vi "Sequencer Main.vi"() -> ()   [LabVIEW 2018] (continued)
              n174 = Greater Than 0?(x=w225) -> (x > 0?=w228:bool)
              n175 = case shown="True" w228 {
                tunnel: w225 -> [_ w233]
                tunnel: [0 w232] -> w227
                frame False {
                }
                frame True {
                  n176 = Decrement(x=w233) -> (x-1=w232:i32)
                }
              }
              n177 = Initialize Array(0, w225) -> (w223:i32[])
              n178 = Greater?(x=w226, y=w227) -> (0:w230:bool)
              n179 = case shown="True" w230 {
                tunnel: w227 -> [_ w235]
                tunnel: w226 -> [w234 _]
                frame False {
                  n180 = local write "Break Point Line"(w234) -> ()
                  n181 = property on="Test Sequencer" class="MCListbox (strict)"("Value"=w234) -> ()  [unwired: 2 in, 2 out]
                }
                frame True {
                  n182 = local write "Break Point Line"(w235) -> ()
                  n183 = property on="Test Sequencer" class="MCListbox (strict)"("Value"=w235) -> ()  [unwired: 2 in, 2 out]
                }
              }
            }
            frame #1 {
              n184 = local read "Break Point Line"() -> (w238:u32)
              n185 = Replace Array Subset(array=w237, new element=1 ("new element/subarray"), index=w238) -> (w239:i32[])
              n186 = global write "Global Variable.vi" "Simbol Array"(w239) -> ()
              n187 = property on="Test Sequencer" class="MCListbox (strict)"("ItemSyms"=w239) -> ()  [unwired: 2 in, 2 out]
            }
          }
        }
        event "Break Point Line": Value Change {
          n188 = event-data() -> ("NewVal"=w241:u32)  [unwired: 1 in, 5 out]
          n189 = flat-sequence {
            tunnel: w241 -> [w245]
            tunnel: [w242] -> w240
            tunnel: w240 -> [w256]
            frame #0 {
              n190 = global read "Sequencer Array.vi" "SEQUENCER Array"() -> (w248:T16[])
              n191 = Array Size(array=w248) -> (size(s)=w244:i32)
              n192 = Greater Than 0?(x=w244) -> (x > 0?=w247:bool)
              n193 = case shown="True" w247 {
                tunnel: w244 -> [_ w252]
                tunnel: [0 w251] -> w246
                frame False {
                }
                frame True {
                  n194 = Decrement(x=w252) -> (x-1=w251:i32)
                }
              }
              n195 = Initialize Array(0, w244) -> (w242:i32[])
              n196 = Greater?(x=w245, y=w246) -> (0:w249:bool)
              n197 = case shown="True" w249 {
                tunnel: w246 -> [_ w254]
                tunnel: w245 -> [w253 _]
                frame False {
                  n198 = local write "Break Point Line"(w253) -> ()
                  n199 = property on="Test Sequencer" class="MCListbox (strict)"("Value"=w253) -> ()  [unwired: 2 in, 2 out]
                }
                frame True {
                  n200 = local write "Break Point Line"(w254) -> ()
                  n201 = property on="Test Sequencer" class="MCListbox (strict)"("Value"=w254) -> ()  [unwired: 2 in, 2 out]
                }
              }
            }
            frame #1 {
              n202 = local read "Break Point Line"() -> (w257:u32)
              n203 = Replace Array Subset(array=w256, new element=1 ("new element/subarray"), index=w257) -> (w258:i32[])
              n204 = global write "Global Variable.vi" "Simbol Array"(w258) -> ()
              n205 = property on="Test Sequencer" class="MCListbox (strict)"("ItemSyms"=w258) -> ()  [unwired: 2 in, 2 out]
            }
          }
        }
        event "Abort Test": Value Change {
          n206 = event-data() -> ()  [unwired: 1 in, 6 out]
          n207 = local read "Debugging"() -> (w261:bool)
          n208 = case shown="True" w261 {
            tunnel: w263 -> [w265 w282]
            tunnel: w262 -> [w266 w281]
            frame False {
              # "!!!!Test Steps Must-be more then 2"
              n209 = global read "Global Variable.vi" "Steps Nmb"() -> (w269:u32)
              n210 = Greater Or Equal?(x=w269, y=u32 2) -> (x >= y?=w268:bool)
              n211 = case shown="True" w268 {
                tunnel: w266 -> [_ w277]
                tunnel: w265 -> [_ w276]
                frame False {
                }
                frame True {
                  w273 = T14 {"Row"=0, "Column"=0} ("Top Left Visible Cell")
                  n212 = global read "Global Variable.vi" "Steps Nmb"() -> (w272:u32)
                  n213 = Subtract(x=w272, y=u32 1) -> (x-y=w271:u32)
                  n214 = Flush Queue(queue=w276, error in (no error)=w277) -> (queue out=w279:refnum<queue>, error out=w278:errorcluster)  [unwired: 1 out]
                  n215 = Enqueue Element(queue=w279, element=w271, error in (no error)=w278) -> ()  [unwired: 1 in, 3 out]
                  n216 = global read "Global Variable.vi" "Report Step Nmb"() -> (w270:u32)
                  n217 = Bundle By Name(cluster=w273, "Row"=w271) -> (w275:T14)
                  n218 = Bundle By Name(cluster=w273, "Row"=w270) -> (w274:T14)
                  n219 = property on="Test Sequencer Run" class="MCListbox (strict)"("TopLeft"=w274) -> ()  [unwired: 2 in, 2 out]
                  n220 = property on="Test Sequencer" class="MCListbox (strict)"("TopLeft"=w275) -> ()  [unwired: 2 in, 2 out]
                }
              }
              n221 = local read "Auto\nRestart"() -> (w264:u16)
              n222 = local write "Restart Cnt"(w264) -> ()
            }
            frame True {
              n223 = flat-sequence {
                tunnel: w282 -> [w290]
                tunnel: w281 -> [w289]
                frame #0 {
                  n224 = global read "Global Variable.vi" "Steps Nmb"() -> (w286:u32)
                  n225 = global read "Global Variable.vi" "Current Step Nmb"() -> (w284:u32)
                  n226 = Decrement(x=w286) -> (x-1=w285:u32)
                  n227 = Greater?(x=w285, y=w284) -> (0:w283:bool)
                  n228 = case shown="True" w283 {
                    frame False {
                    }
                    frame True {
                      n229 = local write "Message"("!!! TEST ABORTED By USER" ("Message")) -> ()
                    }
                  }
                }
                frame #1 {
                  n230 = global read "Global Variable.vi" "Steps Nmb"() -> (w293:u32)
                  n231 = Flush Queue(queue=w290, error in (no error)=w289) -> (queue out=w291:refnum<queue>, error out=w292:errorcluster)  [unwired: 1 out]
                  n232 = local read "Auto\nRestart"() -> (w288:u16)
                  n233 = Decrement(x=w293) -> (x-1=w294:u32)
                  n234 = Enqueue Element(queue=w291, element=w294, error in (no error)=w292) -> ()  [unwired: 1 in, 3 out]
                  n235 = global write "Global Variable.vi" "Current Step Nmb"(w294) -> ()
                  n236 = local write "Restart Cnt"(w288) -> ()
                }
              }
            }
          }
          n237 = global write "Global Variable.vi" "Test Gen Status"(FALSE ("Test Gen Status")) -> ()
          n238 = global write "Global Variable.vi" "System Status"(T1."STOP Sequencer" ("System Status")) -> ()
        }
        event "Load Sequenser": Value Change {
          n239 = event-data() -> ()  [unwired: 1 in, 6 out]
          n240 = global write "Global Variable.vi" "Active Lines Cnt"(u32 0 ("Active Lines Cnt")) -> ()
          n241 = global write "Global Variable.vi" "Report Step Nmb"(u32 0 ("Report Step Nmb")) -> ()
          n242 = control-ref of="Test Sequencer"() -> (w297:refnum<vi>)
          n243 = property on="Tab Edit/Run" class="TabCtl (strict)"("Value"=enum32{"Edit", "Run"}."Edit" ("Tab Edit/Run")) -> ()  [unwired: 2 in, 2 out]
          n244 = in-place {
            in-place-border: w297 -> [w326]
            # "Set Color of all Row to White (Devices)"
            n245 = for {
              N: 250 -> [_]
              tunnel: w326 -> [w328]
              i -> [w329]
              n246 = for {
                N: 10 -> [_]
                tunnel: w329 -> [w334]
                tunnel: w328 -> [w331]
                i -> [w335]
                n247 = Bundle By Name(cluster=T15 {"Row"=0, "Column"=0} ("Active Cell:Active Cell"), "Row"=w334, "Column"=w335) -> (w333:T15)
                n248 = property on="Property Node" class="MCListbox (strict)"(reference=w331, "ActiveCell"=w333, "CellBG"=u32 14013909) -> ()  [unwired: 1 in, 2 out]
              }
            }
          }
          n249 = in-place "In Place Element Structure" {
            in-place-border: w297 -> [w319]
            # "Cleare Sequencer Table"
            n250 = Initialize Array("", 250 ("dimension size"), 10 ("dimension size")) -> (w323:string[][])
            n251 = property on="Property Node" class="MCListbox (strict)"(reference=w319, "ItemNames"=w323, "TopLeft"=T14 {"Row"=0, "Column"=0} ("Top Left Visible Cell"), "Value"=T11 0 ("Test Sequencer")) -> ()  [unwired: 1 in, 2 out]
          }
          n252 = control-ref of="Test Sequencer Run"() -> (w296:refnum<vi>)
          n253 = in-place {
            in-place-border: w296 -> [w308]
            # "Set Color of all Row on Report Table"
            n254 = for {
              N: 250 -> [_]
              tunnel: w308 -> [w310]
              i -> [w311]
              n255 = for {
                N: 7 -> [_]
                tunnel: w311 -> [w316]
                tunnel: w310 -> [w313]
                i -> [w317]
                n256 = Bundle By Name(cluster=T15 {"Row"=0, "Column"=0} ("Active Cell:Active Cell"), "Row"=w316, "Column"=w317) -> (w315:T15)
                n257 = property on="Property Node" class="MCListbox (strict)"(reference=w313, "ActiveCell"=w315, "CellBG"=u32 16448250) -> ()  [unwired: 1 in, 2 out]
              }
            }
          }
          n258 = in-place "In Place Element Structure" {
            in-place-border: w296 -> [w301]
            # "Cleare Sequencer Report Table"
            n259 = Initialize Array("", 250 ("dimension size"), 7 ("dimension size")) -> (w305:string[][])
            n260 = property on="Property Node" class="MCListbox (strict)"(reference=w301, "ItemNames"=w305, "TopLeft"=T14 {"Row"=0, "Column"=0} ("Top Left Visible Cell"), "Value"=T11 0 ("Test Sequencer")) -> ()  [unwired: 1 in, 2 out]
          }
          n261 = global write "Global Variable.vi" "System Status"(T1."INI Secuencer" ("System Status")) -> ()
        }
        event "Button Next Step": Value Change {
          n262 = event-data() -> ()  [unwired: 1 in, 6 out]
          n263 = global read "Global Variable.vi" "Steps Nmb"() -> (w341:u32)
          n264 = global read "Global Variable.vi" "Current Step Nmb"() -> (w340:u32)
          n265 = Decrement(x=w341) -> (x-1=w339:u32)
          n266 = Equal?(x=w339, y=w340) -> (x = y?=w342:bool)
          n267 = case shown="False" w342 {
            tunnel: w338 -> [w345 _]
            tunnel: w337 -> [w344 _]
            frame False {
              n268 = global read "Global Variable.vi" "Current Step Nmb"() -> (w349:u32)
              n269 = Flush Queue(queue=w345, error in (no error)=w344) -> (queue out=w348:refnum<queue>, error out=w347:errorcluster)  [unwired: 1 out]
              n270 = Increment(x=w349) -> (x+1=w346:u32)
              n271 = global write "Global Variable.vi" "Current Step Nmb"(w346) -> ()
              n272 = Enqueue Element(queue=w348, element=w346, error in (no error)=w347) -> ()  [unwired: 1 in, 3 out]
              n273 = global write "Global Variable.vi" "System Status"(T1."START Sequencer" ("System Status")) -> ()
            }
            frame True {
              n274 = global write "Global Variable.vi" "System Status"(T1."Idle" ("System Status")) -> ()
            }
          }
        }
        event "Button Retest": Value Change {
          n275 = event-data() -> ()  [unwired: 1 in, 6 out]
          n276 = global read "Global Variable.vi" "Steps Nmb"() -> (w355:u32)
          n277 = global read "Global Variable.vi" "Current Step Nmb"() -> (w354:u32)
          n278 = Decrement(x=w355) -> (x-1=w353:u32)
          n279 = Equal?(x=w353, y=w354) -> (x = y?=w356:bool)
          n280 = case shown="False" w356 {
            tunnel: w352 -> [w360 _]
            tunnel: w351 -> [w359 _]
            frame False {
              n281 = global read "Global Variable.vi" "Current Step Nmb"() -> (w358:u32)
              n282 = Flush Queue(queue=w360, error in (no error)=w359) -> (queue out=w362:refnum<queue>, error out=w361:errorcluster)  [unwired: 1 out]
              n283 = global write "Global Variable.vi" "Current Step Nmb"(w358) -> ()
              n284 = Enqueue Element(queue=w362, element=w358, error in (no error)=w361) -> ()  [unwired: 1 in, 3 out]
              n285 = global write "Global Variable.vi" "System Status"(T1."START Sequencer" ("System Status")) -> ()
            }
            frame True {
              n286 = global write "Global Variable.vi" "System Status"(T1."Idle" ("System Status")) -> ()
            }
          }
        }
        event "Reset cnt": Value Change {
          w364 = 0
          n287 = event-data() -> ()  [unwired: 1 in, 6 out]
          n288 = local write "Cnt Total"(w364) -> ()
          n289 = local write "Cnt Pass"(w364) -> ()
          n290 = local write "Cnt False"(w364) -> ()
        }
        event "Sequenser": Value Change {
          n291 = event-data() -> ("NewVal"=w367:u16)  [unwired: 1 in, 5 out]
          n292 = global read "Global Variable.vi" "Sequencer Path"() -> (w368:path[])
          n293 = Index Array(array=w368, index=w367) -> (element=w365:path)
          n294 = call-poly <userlib>:"File Exists__ogtk.vi"("file path"=w365) -> ("exists"=w366:bool)  [unwired: 6 in, 1 out]
          n295 = case shown="True" w366 {
            tunnel: w365 -> [_ w372]
            frame False {
            }
            frame True {
              n296 = call <vilib>:"Set Busy.vi"() -> ("error out"=w371:errorcluster)  [unwired: 10 in, 1 out]
              n297 = flat-sequence {
                tunnel: w371 -> [w375]
                tunnel: [w375] -> w370
                tunnel: [w425] -> w374
                tunnel: [w424] -> w373
                tunnel: w372 -> [w422]
                tunnel: w370 -> [w421]
                tunnel: [w421] -> w369
                tunnel: w374 -> [w521]
                tunnel: w373 -> [w520]
                tunnel: w369 -> [w518]
                frame #0 {
                  n298 = global read "Sequencer Array.vi" "SEQUENCER Array"() -> (w378:T16[])
                  n299 = global write "Global Variable.vi" "Steps Cnt"(0) -> ()
                  n300 = control-ref of="Test Sequencer"() -> (w384:refnum<vi>)
                  n301 = global write "Global Variable.vi" "Active Lines Cnt"(u32 0 ("Active Lines Cnt")) -> ()
                  n302 = global write "Global Variable.vi" "Report Step Nmb"(u32 0 ("Report Step Nmb")) -> ()
                  n303 = property on="Tab Edit/Run" class="TabCtl (strict)"("Value"=enum32{"Edit", "Run"}."Edit" ("Tab Edit/Run")) -> ()  [unwired: 2 in, 2 out]
                  n304 = in-place {
                    in-place-border: w384 -> [w403]
                    # "Set Color of all Row to White (Devices)"
                    n305 = for {
                      N: 250 -> [_]
                      tunnel: w403 -> [w405]
                      i -> [w406]
                      n306 = for {
                        N: 10 -> [_]
                        tunnel: w406 -> [w411]
                        tunnel: w405 -> [w408]
                        i -> [w412]
                        n307 = Bundle By Name(cluster=T15 {"Row"=0, "Column"=0} ("Active Cell:Active Cell"), "Row"=w411, "Column"=w412) -> (w410:T15)
                        n308 = property on="Property Node" class="MCListbox (strict)"(reference=w408, "ActiveCell"=w410, "CellBG"=u32 14013909) -> ()  [unwired: 1 in, 2 out]
                      }
                    }
                  }
                  n309 = Array Size(array=w378) -> (size(s)=w377:i32)
                  n310 = in-place "In Place Element Structure" {
                    in-place-border: w384 -> [w414]
                    # "Cleare Sequencer Table"
                    n311 = Initialize Array("", 250 ("dimension size"), 10 ("dimension size")) -> (w418:string[][])
                    n312 = property on="Property Node" class="MCListbox (strict)"(reference=w414, "ItemNames"=w418, "TopLeft"=T14 {"Row"=0, "Column"=0} ("Top Left Visible Cell"), "Value"=T11 0 ("Test Sequencer")) -> ()  [unwired: 1 in, 2 out]
                  }
                  n313 = Delete From Array(array=w378, length=w377) -> (array with subset deleted=w376:T16[])  [unwired: 1 in, 1 out]
                  n314 = global write "Sequencer Array.vi" "SEQUENCER Array"(w376) -> ()
                  n315 = control-ref of="Test Sequencer Run"() -> (w380:refnum<vi>)
                  n316 = in-place "In Place Element Structure" {
                    in-place-border: w380 -> [w396]
                    # "Cleare Sequencer Report Table"
                    n317 = Initialize Array("", 250 ("dimension size"), 7 ("dimension size")) -> (w400:string[][])
                    n318 = property on="Property Node" class="MCListbox (strict)"(reference=w396, "ItemNames"=w400, "TopLeft"=T14 {"Row"=0, "Column"=0} ("Top Left Visible Cell"), "Value"=T11 0 ("Test Sequencer")) -> ()  [unwired: 1 in, 2 out]
                  }
                  n319 = in-place {
                    in-place-border: w380 -> [w385]
                    # "Set Color of all Row on Report Table"
                    n320 = for {
                      N: 250 -> [_]
                      tunnel: w385 -> [w387]
                      i -> [w388]
                      n321 = for {
                        N: 7 -> [_]
                        tunnel: w388 -> [w393]
                        tunnel: w387 -> [w390]
                        i -> [w394]
                        n322 = Bundle By Name(cluster=T15 {"Row"=0, "Column"=0} ("Active Cell:Active Cell"), "Row"=w393, "Column"=w394) -> (w392:T15)
                        n323 = property on="Property Node" class="MCListbox (strict)"(reference=w390, "ActiveCell"=w392, "CellBG"=u32 16448250) -> ()  [unwired: 1 in, 2 out]
                      }
                    }
                  }
                }
                frame #1 {
                  n324 = call <vilib>:"Open Config Data.vi"("create file if necessary (T)"=FALSE, "configuration file path"=w422) -> ("error out"=w429:errorcluster, "refnum"=w430:T19)  [unwired: 7 in, 1 out]
                  n325 = global write "Global Variable.vi" "Steps Cnt"(u16 0 ("Steps Cnt")) -> ()
                  n326 = call <vilib>:"Get Section Names.vi"("error in (no error)"=w429, "refnum"=w430) -> ("error out"=w427:errorcluster, "section names"=w428:string[], "refnum out"=w426:T19)  [unwired: 7 in]
                  n327 = for {
                    tunnel: w428 -> [w436] mode=indexing
                    tunnel: w427 -> [w441]
                    tunnel: w426 -> [w440]
                    tunnel: [w433] -> w425
                    tunnel: [w432] -> w424
                    n328 = Equal?(x=w436, y="Info") -> (x = y?=w442:bool)
                    n329 = case shown="True" w442 {
                      tunnel: w441 -> [w499 w505]
                      tunnel: w440 -> [w500 w504]
                      tunnel: [w500 w503] -> w435
                      tunnel: [w499 w502] -> w434
                      frame False {
                      }
                      frame True {
                        w516 = "***"
                        w512 = "Info"
                        n330 = call-poly <vilib>:"Read Key.vi"("section"=w512, "error in (no error)"=w505, "default value"=w516, "key"="Customer", "refnum"=w504) -> ("error out"=w509:errorcluster, "value"=w501:string, "refnum out"=w511:T19)  [unwired: 3 in, 1 out]
                        n331 = call-poly <vilib>:"Read Key.vi"("section"=w512, "error in (no error)"=w509, "default value"=w516, "key"="Board", "refnum"=w511) -> ("error out"=w508:errorcluster, "value"=w507:string, "refnum out"=w510:T19)  [unwired: 3 in, 1 out]
                        n332 = call-poly <vilib>:"Read Key.vi"("section"=w512, "error in (no error)"=w508, "default value"=w516, "key"="Config", "refnum"=w510) -> ("error out"=w502:errorcluster, "value"=w506:string, "refnum out"=w503:T19)  [unwired: 3 in, 1 out]
                        n333 = global write "Global Variable.vi" "Customer"(w501) -> ()
                        n334 = global write "Global Variable.vi" "Config"(w506) -> ()
                        n335 = global write "Global Variable.vi" "Board"(w507) -> ()
                      }
                    }
                    n336 = Match Pattern(string=w436, regular expression="Step") -> (offset past match=w439:i32)  [unwired: 1 in, 3 out]
                    n337 = Greater Or Equal To 0?(x=w439) -> (x >= 0?=w437:bool)
                    n338 = case shown="True" w437 {
                      tunnel: w436 -> [_ w463]
                      tunnel: w435 -> [w445 w462]
                      tunnel: w434 -> [w444 w461]
                      tunnel: [w445 w449] -> w433
                      tunnel: [w444 w448] -> w432
                      frame False {
                      }
                      frame True {
                        n339 = call-poly <vilib>:"Read Key.vi"("section"=w463, "error in (no error)"=w461, "key"="Step ID", "refnum"=w462) -> ("error out"=w466:errorcluster, "value"=w460:u32, "refnum out"=w465:T19)  [unwired: 4 in, 1 out]
                        n340 = call-poly <vilib>:"Read Key.vi"("section"=w463, "error in (no error)"=w466, "key"="Description", "refnum"=w465) -> ("error out"=w470:errorcluster, "value"=w459:string, "refnum out"=w469:T19)  [unwired: 4 in, 1 out]
                        n341 = call-poly <vilib>:"Read Key.vi"("section"=w463, "error in (no error)"=w470, "key"="Step Type", "refnum"=w469) -> ("error out"=w473:errorcluster, "value"=w458:u32, "refnum out"=w472:T19)  [unwired: 4 in, 1 out]
                        n342 = call-poly <vilib>:"Read Key.vi"("section"=w463, "error in (no error)"=w473, "key"="Measurement Units", "refnum"=w472) -> ("error out"=w477:errorcluster, "value"=w457:string, "refnum out"=w474:T19)  [unwired: 4 in, 1 out]
                        n343 = call-poly <vilib>:"Read Key.vi"("section"=w463, "error in (no error)"=w477, "key"="Nominal Value", "refnum"=w474) -> ("error out"=w478:errorcluster, "value"=w456:dbl, "refnum out"=w475:T19)  [unwired: 4 in, 1 out]
                        n344 = global read "Global Variable.vi" "Steps Cnt"() -> (w446:u16)
                        n345 = call-poly <vilib>:"Read Key.vi"("section"=w463, "error in (no error)"=w478, "key"="Upper Value", "refnum"=w475) -> ("error out"=w479:errorcluster, "value"=w455:dbl, "refnum out"=w476:T19)  [unwired: 4 in, 1 out]
                        n346 = Increment(x=w446) -> (x+1=w447:u16)
                        n347 = call-poly <vilib>:"Read Key.vi"("section"=w463, "error in (no error)"=w479, "key"="Lower Value", "refnum"=w476) -> ("error out"=w484:errorcluster, "value"=w454:dbl, "refnum out"=w483:T19)  [unwired: 4 in, 1 out]
                        n348 = global write "Global Variable.vi" "Steps Cnt"(w447) -> ()
                        n349 = call-poly <vilib>:"Read Key.vi"("section"=w463, "error in (no error)"=w484, "key"="Parameters", "refnum"=w483) -> ("error out"=w489:errorcluster, "value"=w453:string, "refnum out"=w486:T19)  [unwired: 4 in, 1 out]
                        n350 = call-poly <vilib>:"Read Key.vi"("section"=w463, "error in (no error)"=w489, "key"="Run/Skip", "refnum"=w486) -> ("error out"=w490:errorcluster, "value"=w452:bool, "refnum out"=w487:T19)  [unwired: 4 in, 1 out]
                        n351 = call-poly <vilib>:"Read Key.vi"("section"=w463, "error in (no error)"=w490, "key"="Report", "refnum"=w487) -> ("error out"=w491:errorcluster, "value"=w451:bool, "refnum out"=w488:T19)  [unwired: 4 in, 1 out]
                        n352 = call-poly <vilib>:"Read Key.vi"("section"=w463, "error in (no error)"=w491, "key"="Test Result", "refnum"=w488) -> ("error out"=w448:errorcluster, "value"=w450:u32, "refnum out"=w449:T19)  [unwired: 4 in, 1 out]
                        n353 = Bundle By Name(cluster=T16 {"Step ID"=0, "Step Description"="", "Step Type"=0, "Test Values"={"Numeric Value"=0.0, "Str Value"="", "Boolean Value"=TRUE, "Upper Limit"=0.0, "Lower Limit"=0.0}, "Parameters"="", "Run/Skip"=TRUE, "Test Result"=enum."Idle", "Report"=TRUE, "Measure Units"="..."} ("Test Step"), "Step ID"=w460, "Step Description"=w459, "Step Type"=w458, "Measure Units"=w457, "Test Values.Numeric Value"=w456, "Test Values.Upper Limit"=w455, "Test Values.Lower Limit"=w454, "Parameters"=w453, "Run/Skip"=w452, "Report"=w451, "Test Result"=w450) -> (w498:T16)
                        n354 = global read "Sequencer Array.vi" "SEQUENCER Array"() -> (w495:T16[])
                        n355 = Insert Into Array(array=w495, index=w446, new element=w498) -> (w496:T16[])
                        n356 = global write "Sequencer Array.vi" "SEQUENCER Array"(w496) -> ()
                      }
                    }
                  }
                }
                frame #2 {
                  n357 = in-place {
                    n358 = global write "Global Variable.vi" "System Status"(T1."INI Secuencer" ("System Status")) -> ()
                  }
                  n359 = call <vilib>:"Unset Busy.vi"("error in (no error)"=w518) -> ("error out"=w517:errorcluster)  [unwired: 10 in]
                  n360 = call <vilib>:"Close Config Data.vi"("error in (no error)"=w520, "write file if changed (T)"=TRUE, "refnum"=w521) -> ("error out"=w523:errorcluster)  [unwired: 7 in, 1 out]
                  n361 = call <userlib>:"Clear All Errors__ogtk.vi"("Error In"=w517) -> ()  [unwired: 3 in, 1 out]
                  n362 = call <vilib>:"Simple Error Handler.vi"("error in (no error)"=w523) -> ()  [unwired: 4 in, 5 out]
                  n363 = property on="Tab Control Main" class="TabCtl (strict)"("Value"=T2."TEST Board" ("Tab Control Main")) -> ()  [unwired: 2 in, 2 out]
                }
              }
            }
          }
        }
      }
    }
  }
  n364 = in-place {
    in-place-border: w5 -> [w528]
    in-place-border: w4 -> [w527]
    in-place-border: w3 -> [w526]
    in-place-border: w2 -> [w525]
    n365 = while {
      tunnel: w528 -> [w532]
      tunnel: w527 -> [w531]
      tunnel: w526 -> [w530]
      tunnel: w525 -> [w529]
      stop <- FALSE stop-if-true
      # "250"
      # "READ System GPIO"
      n366 = event shown="[0] Timeout" {
        selector: _ -> [_]
        dyn-events: _ -> [_]
        timeout: 50 -> [_]
        tunnel: w532 -> [w539]
        tunnel: w531 -> [w540]
        tunnel: w530 -> [w536]
        tunnel: w529 -> [w535]
        event Timeout {
          n367 = event-data() -> ()  [unwired: 1 in, 3 out]
          n368 = call <vilib>:"Acquire Semaphore.vi"("error in (no error)"=w539, "semaphore"=w540) -> ("error out"=w538:errorcluster, "semaphore out"=w537:T13)  [unwired: 3 in, 1 out]
          n369 = case shown="No Error" w538 {
            selector: w538 -> [w557 _]
            tunnel: w537 -> [w556 _]
            tunnel: w536 -> [w555 _]
            tunnel: w535 -> [w554 _]
            frame No Error {
              n370 = flat-sequence {
                tunnel: w557 -> [w559]
                tunnel: w556 -> [w558]
                tunnel: w555 -> [w588]
                tunnel: [w588] -> w553
                tunnel: w554 -> [w593]
                tunnel: [w593] -> w552
                tunnel: [w580] -> w551
                tunnel: [w578] -> w550
                tunnel: [w576] -> w549
                tunnel: [w575] -> w548
                tunnel: [w564] -> w543
                tunnel: [w559] -> w542
                tunnel: [w558] -> w541
                tunnel: w553 -> [w653]
                tunnel: [w653] -> w547
                tunnel: w552 -> [w652]
                tunnel: [w652] -> w546
                tunnel: [w649] -> w545
                tunnel: w551 -> [w650]
                tunnel: w550 -> [w644]
                tunnel: w549 -> [w645]
                tunnel: w548 -> [w651]
                tunnel: [w647] -> w544
                tunnel: w543 -> [w648]
                tunnel: w542 -> [w643]
                tunnel: w541 -> [w642]
                tunnel: w544 -> [w660]
                tunnel: w545 -> [w662]
                tunnel: w546 -> [w663]
                tunnel: w547 -> [w661]
                frame #0 {
                  w602 = T20 7 items=["Addr-0"=0, "Addr-1"=4, "Addr-2"=2, "Addr-3"=6, "Addr-4"=1, "Addr-5"=5, "Addr-6"=3, "Addr-7"=7] ("Addr")
                  # "DigIn 3"
                  # "ReSTART"
                  # "no dio err"
                  # "Stop AUTO"
                  # "Start AUTO"
                  # "Start Button"
                  # "Stop Button"
                  # "READ SYS Dig In"
                  n371 = global read "Global Variable.vi" "FTDI SPI Handle"() -> (w603:u32)
                  n372 = in-place {
                    in-place-border: [w631] -> _
                    in-place-border: [w630] -> w592
                    n373 = property on="Tab Control Main" class="TabCtl (strict)"() -> ("Value"=w629:T2)  [unwired: 2 in, 2 out]
                    n374 = property on="Run Test" class="Bool"() -> ("DisabledEnum"=w632:T18)  [unwired: 2 in, 2 out]
                    n375 = case shown="\"Enabled\", Default" w632 {
                      tunnel: [TRUE FALSE FALSE] -> w631
                      frame "Enabled", Default {
                      }
                      frame "Disabled and Grayed Out" {
                      }
                      frame "Disabled" {
                      }
                    }
                    n376 = case shown="\"TEST Board\"" w629 {
                      tunnel: [FALSE TRUE] -> w630
                      frame "INI System", Default {
                      }
                      frame "TEST Board" {
                      }
                    }
                  }
                  n377 = call "FTDI SPI SYS Read.vi"("nCS"=u8 2, "Use Extra"=TRUE, "Addr"=w602, "Handler In"=w603) -> ("Out Reg B Bin"=w601:bool[])  [unwired: 2 in, 5 out]
                  n378 = Index Array(array=w601, index #1=0 ("index"), index #2=1 ("index"), index #3=2 ("index"), index #4=3 ("index"), index #5=4 ("index")) -> (element #1=w568:bool, element #2=w590:bool, element #3=w569:bool, element #4=w563:bool, element #5=w594:bool)
                  n379 = local read "Auto\nReStart"() -> (w565:bool)
                  n380 = feedback #1() -> (w589:bool)  [unwired: 1 in]
                  n381 = Not(x=w589) -> (.not. x?=w584:bool)
                  n382 = local read "Dig-IN Claster"() -> (w595:T12)
                  n383 = Not(x=w568) -> (.not. x?=w570:bool)
                  n384 = And(x=w568, y=w590) -> (x .and. y?=w562:bool)
                  n385 = feedback-in #1(w562) -> ()
                  n386 = Bundle By Name(cluster=w595, "Stop"=w590, "Fixture Close"=w569, "digIn 3"=w563, "digIn 4"=w594, "Run"=w568) -> (w572:T12)
                  n387 = in-place {
                    in-place-border: TRUE -> [w627]
                    in-place-border: w592 -> [w626]
                    in-place-border: w568 -> [w625]
                    in-place-border: [w624] -> w579
                    # "Run"
                    n388 = feedback #2() -> (w628:bool)  [unwired: 1 in]
                    n389 = feedback-in #2(w625) -> ()
                    n390 = Compound Arithmetic op=AND(invert w625, w628, w626, w627) -> (w624:bool)
                  }
                  n391 = in-place {
                    in-place-border: w590 -> [w613]
                    in-place-border: w562 -> [w611]
                    in-place-border: [w610] -> w581
                    # "Stop"
                    n392 = feedback #3() -> (w612:bool)  [unwired: 1 in]
                    n393 = feedback-in #3(w613) -> ()
                    n394 = Compound Arithmetic op=AND(w613, w612, invert w611) -> (w610:bool)
                  }
                  n395 = And(x=w570, y=w569) -> (x .and. y?=w571:bool)
                  n396 = case shown="False" w584 {
                    frame False {
                      n397 = property on="Sys Err" class="Bool (strict)"() -> ("Value"=w639:bool)  [unwired: 2 in, 2 out]
                      n398 = Compound Arithmetic op=AND(TRUE ("value"), invert w639) -> (w640:bool)
                      n399 = property on="Sys Err" class="Bool (strict)"("Value"=w640) -> ()  [unwired: 2 in, 2 out]
                    }
                    frame True {
                      n400 = property on="Sys Err" class="Bool (strict)"("Value"=FALSE ("Sys Err")) -> ()  [unwired: 2 in, 2 out]
                    }
                  }
                  n401 = global write "Global Variable.vi" "Sys ERR"(w562) -> ()
                  n402 = case shown="True" "Auto\nSTART" {
                    tunnel: [w614 w617] -> w577
                    tunnel: [w614 w616] -> w574
                    tunnel: w571 -> [_ w615]
                    frame False {
                      w614 = FALSE
                    }
                    frame True {
                      n403 = in-place {
                        in-place-border: w615 -> [w623]
                        in-place-border: [w621] -> w616
                        # "STOP Condition"
                        n404 = feedback #4() -> (w622:bool)  [unwired: 1 in]
                        n405 = feedback-in #4(w623) -> ()
                        n406 = Compound Arithmetic op=AND(invert w623, w622) -> (w621:bool)
                      }
                      n407 = in-place {
                        in-place-border: w615 -> [w620]
                        in-place-border: [w618] -> w617
                        # "START Condition"
                        n408 = feedback #5() -> (w619:bool)  [unwired: 1 in]
                        n409 = feedback-in #5(w620) -> ()
                        n410 = Compound Arithmetic op=AND(w620, invert w619) -> (w618:bool)
                      }
                    }
                  }
                  n411 = local write "Dig-IN Claster"(w572) -> ()
                  n412 = global read "Global Variable.vi" "System Status"() -> (w583:T1)
                  n413 = global read "Global Variable.vi" "System Status"() -> (w586:T1)
                  n414 = Equal?(x=w583, y=T1."Idle" ("System Status")) -> (x = y?=w566:bool)
                  n415 = Equal?(x=w586, y=T1."Run Sequencer" ("System Status")) -> (x = y?=w573:bool)
                  n416 = case shown="\"Idle\"" T1."Idle" ("System Status") {
                    tunnel: w563 -> [w604 _]
                    frame "Idle" {
                      # "Reset Barcode"
                      n417 = in-place {
                        in-place-border: w604 -> [w609]
                        in-place-border: [w607] -> w605
                        # "Barcode\nrst"
                        n418 = feedback #6() -> (w608:bool)  [unwired: 1 in]
                        n419 = feedback-in #6(w609) -> ()
                        n420 = Compound Arithmetic op=AND(w609, invert w608) -> (w607:bool)
                      }
                      n421 = case shown="True" w605 {
                        frame False {
                        }
                        frame True {
                          n422 = global write "Global Variable.vi" "Reset BARCODE"(TRUE ("Reset BARCODE")) -> ()
                        }
                      }
                    }
                    frame "INI System", Default {
                    }
                  }
                  n423 = And(x=w565, y=w566) -> (x .and. y?=w564:bool)
                  n424 = And(x=w577, y=w566) -> (x .and. y?=w576:bool)
                  n425 = And(x=w573, y=w581) -> (x .and. y?=w580:bool)
                  n426 = And(x=w566, y=w579) -> (x .and. y?=w578:bool)
                  n427 = And(x=w574, y=w573) -> (x .and. y?=w575:bool)
                }
                frame #1 {
                  # "Run"
                  # "Stop"
                  # "Auto RESTART"
                  n428 = call <vilib>:"Release Semaphore.vi"("error in (no error)"=w643, "semaphore"=w642) -> ()  [unwired: 4 in, 2 out]
                  n429 = Or(x=w651, y=w650) -> (x .or. y?=w649:bool)
                  n430 = Compound Arithmetic op=OR(w648, w645, w644) -> (w647:bool)
                  n431 = case shown="True" w649 {
                    frame False {
                    }
                    frame True {
                      # "No Report Generation"
                      n432 = local read "Auto\nRestart"() -> (w657:u16)
                      n433 = global write "Global Variable.vi" "Cancel by operator"(TRUE ("Cancel by operator")) -> ()
                      n434 = global write "Global Variable.vi" "Test Gen Status"(FALSE ("Test Gen Status")) -> ()
                      n435 = local write "Restart Cnt"(w657) -> ()
                      n436 = global write "Global Variable.vi" "System Status"(T1."STOP Sequencer" ("System Status")) -> ()
                    }
                  }
                  n437 = case shown="True" w647 {
                    frame False {
                    }
                    frame True {
                      n438 = global write "Global Variable.vi" "System Status"(T1."START Sequencer" ("System Status")) -> ()
                    }
                  }
                  n439 = Or(x=w645, y=w644) -> (x .or. y?=w646:bool)
                  n440 = case shown="True" w646 {
                    frame False {
                    }
                    frame True {
                      n441 = local write "Restart Cnt"(u16 0 ("Restart Cnt")) -> ()
                    }
                  }
                }
                frame #2 {
                  # "Stop"
                  # "Run"
                  n442 = case shown="False" w660 {
                    tunnel: w661 -> [w665 w707]
                    tunnel: w663 -> [w664 w706]
                    tunnel: w662 -> [w666 _]
                    frame False {
                      n443 = case shown="True" w666 {
                        tunnel: w665 -> [_ w669]
                        tunnel: w664 -> [_ w668]
                        frame False {
                        }
                        frame True {
                          # "STOP"
                          n444 = local read "Debugging"() -> (w667:bool)
                          n445 = case shown="True" w667 {
                            tunnel: w669 -> [w670 w687]
                            tunnel: w668 -> [w671 w686]
                            frame False {
                              # "!!!!Test Steps Must-be more then 2"
                              n446 = global read "Global Variable.vi" "Steps Nmb"() -> (w674:u32)
                              n447 = Greater Or Equal?(x=w674, y=u32 2) -> (x >= y?=w673:bool)
                              n448 = case shown="True" w673 {
                                tunnel: w671 -> [_ w682]
                                tunnel: w670 -> [_ w681]
                                frame False {
                                }
                                frame True {
                                w678 = T14 {"Row"=0, "Column"=0} ("Top Left Visible Cell")
                                n449 = global read "Global Variable.vi" "Steps Nmb"() -> (w677:u32)
                                n450 = global read "Global Variable.vi" "Report Step Nmb"() -> (w675:u32)
                                n451 = Flush Queue(queue=w681, error in (no error)=w682) -> (queue out=w684:refnum<queue>, error out=w683:errorcluster)  [unwired: 1 out]
                                n452 = Subtract(x=w677, y=u32 1) -> (x-y=w676:u32)
                                n453 = Enqueue Element(queue=w684, element=w676, error in (no error)=w683) -> ()  [unwired: 1 in, 3 out]
                                n454 = Bundle By Name(cluster=w678, "Row"=w676) -> (w680:T14)
                                n455 = Bundle By Name(cluster=w678, "Row"=w675) -> (w679:T14)
                                n456 = property on="Test Sequencer Run" class="MCListbox (strict)"("TopLeft"=w679) -> ()  [unwired: 2 in, 2 out]
                                n457 = property on="Test Sequencer" class="MCListbox (strict)"("TopLeft"=w680) -> ()  [unwired: 2 in, 2 out]
                                }
                              }
                            }
                            frame True {
                              n458 = flat-sequence {
                                tunnel: w687 -> [w694]
                                tunnel: w686 -> [w693]
                                frame #0 {
                                n459 = global read "Global Variable.vi" "Steps Nmb"() -> (w691:u32)
                                n460 = global read "Global Variable.vi" "Current Step Nmb"() -> (w689:u32)
                                n461 = Decrement(x=w691) -> (x-1=w690:u32)
                                n462 = Greater?(x=w690, y=w689) -> (0:w688:bool)
                                n463 = case shown="True" w688 {
                                frame False {
                                }
                                frame True {
                                n464 = local write "Message"("!!! TEST ABORTED By USER" ("Message")) -> ()
                                }
                                }
                                }
                                frame #1 {
                                n465 = global read "Global Variable.vi" "Steps Nmb"() -> (w697:u32)
                                n466 = Flush Queue(queue=w694, error in (no error)=w693) -> (queue out=w695:refnum<queue>, error out=w696:errorcluster)  [unwired: 1 out]
                                n467 = Decrement(x=w697) -> (x-1=w698:u32)
                                n468 = global write "Global Variable.vi" "Current Step Nmb"(w698) -> ()
                                n469 = Enqueue Element(queue=w695, element=w698, error in (no error)=w696) -> ()  [unwired: 1 in, 3 out]
                                }
                              }
                            }
                          }
                        }
                      }
                    }
                    frame True {
                      w699 = u32 0 ("Active Lines Cnt")
                      w710 = u32 0 ("Row")
                      # "START"
                      n470 = Bundle By Name(cluster=T14 {"Row"=0, "Column"=0} ("Top Left Visible Cell"), "Row"=w710) -> (w709:T14)
                      n471 = global read "Sequencer Array.vi" "SEQUENCER Array"() -> (w703:T16[])
                      n472 = global write "Global Variable.vi" "Active Lines Cnt"(w699) -> ()
                      n473 = global write "Global Variable.vi" "Report Active Lines Cnt"(w699) -> ()
                      n474 = global write "Global Variable.vi" "Report Step Nmb"(w699) -> ()
                      n475 = global write "Global Variable.vi" "Test Time"(w699) -> ()
                      n476 = property on="Test Sequencer" class="MCListbox (strict)"("TopLeft"=w709, "Value"=w710) -> ()  [unwired: 2 in, 2 out]
                      n477 = property on="Test Sequencer Run" class="MCListbox (strict)"("TopLeft"=w709, "Value"=w710) -> ()  [unwired: 2 in, 2 out]
                      n478 = local read "Debugging"() -> (w702:bool)
                      n479 = Flush Queue(queue=w707, error in (no error)=w706) -> (queue out=w705:refnum<queue>, error out=w704:errorcluster)  [unwired: 1 out]
                      n480 = Array Size(array=w703) -> (size(s)=w700:i32)
                      n481 = for {
                        N: w700 -> [_]
                        i -> [w744]
                        n482 = property on="Test Squencer Edit" class="MCListbox (strict)"() -> ("ItemNames"=w750:string[][])  [unwired: 2 in, 2 out]
                        n483 = Bundle By Name(cluster=T15 {"Row"=0, "Column"=0} ("Active Cell:Active Cell"), "Row"=w744, "Column"=5) -> (w745:T15)
                        n484 = Replace Array Subset(array=w750, new element="Idle", index (row)=w744, index (col)=5 ("disabled index (col)")) -> (w749:string[][])
                        n485 = property on="Test Squencer Edit" class="MCListbox (strict)"("ItemNames"=w749, "ActiveCell"=w745, "CellFontColor"=u32 16448250) -> ()  [unwired: 2 in, 2 out]
                      }
                      n486 = case shown="False" w702 {
                        tunnel: w705 -> [w731 w738]
                        tunnel: w704 -> [w730 w737]
                        tunnel: w700 -> [w729 _]
                        frame False {
                          n487 = for {
                            N: w729 -> [_]
                            tunnel: w731 -> [w732]
                            tunnel: w730 -> [w734]
                            i -> [w733]
                            n488 = Enqueue Element(queue=w732, element=w733, error in (no error)=w734) -> ()  [unwired: 1 in, 3 out]
                          }
                        }
                        frame True {
                          n489 = local read "Break Point Line"() -> (w735:u32)
                          n490 = Increment(x=w735) -> (x+1=w736:u32)
                          n491 = for {
                            N: w736 -> [_]
                            tunnel: w738 -> [w741]
                            tunnel: w737 -> [w740]
                            i -> [w739]
                            n492 = Enqueue Element(queue=w741, element=w739, error in (no error)=w740) -> ()  [unwired: 1 in, 3 out]
                          }
                        }
                      }
                      n493 = control-ref of="Test Sequencer Run"() -> (w701:refnum<vi>)
                      n494 = in-place "In Place Element Structure" {
                        in-place-border: w701 -> [w712]
                        in-place-border: w700 -> [w711]
                        # "Cleare Sequencer Report Table"
                        n495 = Initialize Array("", w711, 7 ("dimension size")) -> (w716:string[][])
                        n496 = property on="Property Node" class="MCListbox (strict)"(reference=w712, "ItemNames"=w716, "TopLeft"=T14 {"Row"=0, "Column"=0} ("Top Left Visible Cell"), "Value"=T11 0 ("Test Sequencer")) -> ()  [unwired: 1 in, 2 out]
                      }
                      n497 = in-place {
                        in-place-border: w701 -> [w719]
                        in-place-border: w700 -> [w718]
                        # "Set Color of all Row on Report Table"
                        n498 = for {
                          N: w718 -> [_]
                          tunnel: w719 -> [w720]
                          i -> [w721]
                          n499 = for {
                            N: 7 -> [_]
                            tunnel: w721 -> [w726]
                            tunnel: w720 -> [w723]
                            i -> [w727]
                            n500 = Bundle By Name(cluster=T15 {"Row"=0, "Column"=0} ("Active Cell:Active Cell"), "Row"=w726, "Column"=w727) -> (w725:T15)
                            n501 = property on="Property Node" class="MCListbox (strict)"(reference=w723, "ActiveCell"=w725, "CellBG"=u32 16448250) -> ()  [unwired: 1 in, 2 out]
                          }
                        }
                      }
                    }
                  }
                }
              }
            }
            frame Error {
            }
          }
        }
      }
    }
  }
  n502 = in-place {
    in-place-border: w3 -> [w754]
    in-place-border: w2 -> [w753]
    in-place-border: w5 -> [w752]
    in-place-border: w4 -> [w751]
    # "MAIN LOOP SECTION"
    n503 = while {
      tunnel: w754 -> [w759]
      tunnel: w753 -> [w758]
      tunnel: w752 -> [w757]
      tunnel: w751 -> [w756]
      stop <- FALSE stop-if-true
      # "MAIN LOOP"
      n504 = global read "Global Variable.vi" "System Status"() -> (w755:T1)
      "System Status" <- w755
      n505 = case shown="\"INI Devices\"" w755 {
        tunnel: w759 -> [_ _ _ _ _ w1453 _ _ _ _]
        tunnel: w758 -> [_ _ _ _ _ w1456 _ _ _ _]
        tunnel: w757 -> [_ _ _ _ w1366 w1455 w6210 _ _ _]
        tunnel: w756 -> [_ _ _ _ w1367 w1454 w6209 _ _ _]
        frame "Idle" {
          n506 = global read "Global Variable.vi" "Reset BARCODE"() -> (w761:bool)
          n507 = case shown="True" w761 {
            frame False {
            }
            frame True {
              # "? Muve PANNEL to top of Desk"
              n508 = case shown="True" TRUE {
                frame False {
                }
                frame True {
                  n509 = flat-sequence {
                    frame #0 {
                      # "? Muve PANNEL to top of Desk"
                      n510 = case shown="True" FALSE {
                        frame False {
                        }
                        frame True {
                          n511 = vi-ref "PanelOnTop.vi"() -> (w782:refnum<vi>)
                          n512 = property class="VI"(reference=w782) -> (error out=w785:errorcluster, "Name"=w778:string)  [unwired: 1 in, 1 out]
                          n513 = control-ref of="This VI"() -> (w774:refnum<vi>)
                          n514 = Open VI Reference(type specifier VI Refnum (for type only)=refnum<vi> refnum, vi path=w778, options=256, error in (no error)=w785) -> (vi reference=w777:refnum<vi>, error out=w776:errorcluster)  [unwired: 2 in]
                          n515 = call-by-ref "Start Asynchronous Call"(reference=w777, error in=w776, "VI Refnum"=w774) -> ()  [unwired: 8 in, 5 out]
                          n516 = call-by-ref "Wait On Asynchronous Call"(reference=w777, error in=w776) -> (reference out=w780:refnum<vi>, error out=w779:errorcluster, "Handler"=→"Handler":u32)  [unwired: 9 in, 2 out]
                          n517 = Wait (ms)(milliseconds to wait=u32 250) -> ()  [unwired: 1 out]
                          n518 = Close Reference(reference=w780, error in (no error)=w779) -> ()  [unwired: 1 out]
                        }
                      }
                    }
                    frame #1 {
                      n519 = local read "Barcode\nDefault"() -> (w788:bool)
                      n520 = Wait (ms)(milliseconds to wait=u32 50) -> ()  [unwired: 1 out]
                      n521 = case shown="True" w788 {
                        frame False {
                          n522 = property on="Barcode" class="Str"("Value"="", "Key Focus"=TRUE) -> ()  [unwired: 2 in, 2 out]
                        }
                        frame True {
                          n523 = property on="Barcode" class="Str"("Value"="ADB-12345") -> ()  [unwired: 2 in, 2 out]
                        }
                      }
                      n524 = global write "Global Variable.vi" "Reset BARCODE"(FALSE ("Reset BARCODE")) -> ()
                    }
                  }
                }
              }
              n525 = case shown="True" FALSE {
                frame False {
                }
                frame True {
                  n526 = control-ref of="This VI"() -> (w772:refnum<vi>)
                  n527 = call <vilib>:"Application Directory.vi"() -> ("Application Directory"=w764:path)
                  n528 = property class="VI" props=["Front Panel.IsFrontmost"](reference=w772) -> (error out=w768:errorcluster)  [unwired: 1 in, 2 out]
                  n529 = Path To String(path=w764) -> (string=w771:string)
                  n530 = Concatenate Strings(w771, "\\sendkeys.bat \"LabVIEW\"") -> (w769:string)
                  n531 = call <vilib>:"System Exec.vi"("run minimized? (F)"=TRUE, "wait until completion? (T)"=TRUE, "error in (no error)"=w768, "command line"=w769) -> ("error out"=w767:errorcluster)  [unwired: 4 in, 3 out]
                  n532 = call <userlib>:"Clear All Errors__ogtk.vi"("Error In"=w767) -> ()  [unwired: 3 in, 1 out]
                }
              }
            }
          }
        }
        frame "INI System" {
          n533 = flat-sequence {
            tunnel: [w802] -> w792
            tunnel: w792 -> [w905]
            frame #0 {
              w793 = ""
              w794 = 0
              w797 = 0
              w796 = i32[] [0, 0, 0, 0, 0, 0] ("Disabled Items []")
              w795 = string[] ["---", "---", "---", "---", "---", "---"] ("Strings []")
              n534 = local write "Under Test BOARD"(w793) -> ()
              n535 = local write "Customer"(w793) -> ()
              n536 = local write "Config"(w793) -> ()
              n537 = local write "Cnt Pass All"(w797) -> ()
              n538 = local write "Cnt False All"(w797) -> ()
              n539 = local write "Cnt Total All"(w797) -> ()
              n540 = property on="Sequenser" class="Ring (strict)"("Disabled Items []"=w796, "Strings []"=w795, "Value"=w794) -> ()  [unwired: 2 in, 2 out]
              n541 = property on="Operator" class="Ring (strict)"("Disabled Items []"=w796, "Strings []"=w795, "Value"=w794) -> ()  [unwired: 2 in, 2 out]
            }
            frame #1 {
              # "Read INI System File"
              n542 = call <vilib>:"Application Directory.vi"() -> ("Application Directory"=w813:path)
              n543 = Build Path(base path=w813, name or relative path="INI\\SysConfig.ini") -> (appended path=w815:path)
              n544 = call <vilib>:"Check if File or Folder Exists.vi"("path"=w815) -> ("error out"=w811:errorcluster, "dup path"=w803:path)  [unwired: 8 in, 1 out]
              n545 = case shown="No Error" w811 {
                tunnel: w803 -> [_ w904]
                tunnel: [FALSE TRUE] -> w802
                frame Error {
                  n546 = One Button Dialog(message="System INI File Missing!") -> ()  [unwired: 1 in, 1 out]
                }
                frame No Error {
                  "System INI Config File" <- w904
                }
              }
              n547 = call <vilib>:"Open Config Data.vi"("error in (no error)"=w811, "create file if necessary (T)"=FALSE, "configuration file path"=w803) -> ("error out"=w800:errorcluster, "refnum"=w801:T19)  [unwired: 6 in, 1 out]
              n548 = in-place {
                in-place-border: w801 -> [w841]
                in-place-border: w800 -> [w840]
                in-place-border: [w839] -> w799
                in-place-border: [w838] -> w798
                # "Sequencer"
                n549 = for {
                  N: 10 -> [_]
                  shift-right: [w852] -> w839
                  shift-left: w841 -> [w865]
                  shift-right: [w854] -> w838
                  shift-left: w840 -> [w864]
                  i -> [w849]
                  n550 = Number To Decimal String(number=w849) -> (decimal integer string=w861:string)  [unwired: 1 in]
                  n551 = property on="Sequenser" class="Ring (strict)"() -> ("StringsAndValues[]"=w858:T33)  [unwired: 2 in, 2 out]
                  n552 = Concatenate Strings("Sequencer-" ("section"), w861) -> (w846:string)
                  n553 = call-poly <vilib>:"Read Key.vi"("section"=w846, "error in (no error)"=w864, "key"="Name", "refnum"=w865) -> ("value"=w859:string, "refnum out"=w853:T19)  [unwired: 4 in, 2 out]
                  n554 = Index Array(array=w858, index=w849) -> (element=w860:cluster{"String":string, "Value":u16})
                  n555 = global read "Global Variable.vi" "Sequencer Path"() -> (w850:path[])
                  n556 = Bundle By Name(cluster=w860, "String"=w859, "Value"=w849) -> (w857:cluster{"String":string, "Value":u16})
                  n557 = call-poly <vilib>:"Read Key.vi"("section"=w846, "default value"="***", "key"="Directory", "refnum"=w853) -> ("value"=w848:string, "found?"=w843:bool, "refnum out"=w852:T19)  [unwired: 4 in, 1 out]
                  n558 = Replace Array Subset(array=w858, new element=w857, index=w849) -> (w856:T33)
                  n559 = String To Path(string=w848) -> (path=w847:path)
